vi "Serial-Communication-LabVIEW.vi"() -> ()   [LabVIEW 2016]
uses:
  <vilib>/Instr/_visa.llb/VISA Configure Serial Port (Instr).vi
panel:
  out "O7":bool
  out "O6":bool
  out "O5":bool
  out "O4":bool
  out "O3":bool
  out "O2":bool
  out "O1":bool
  out "O0":bool
  in  "17":bool
  in  "16":bool
  in  "15":bool
  in  "14":bool
  in  "13":bool
  in  "12":bool
  in  "11":bool
  in  "10":bool
  in  "stop":bool
  in  "milliseconds to wait":u32
  in  "VISA resource name":refnum<visa-resource-name>
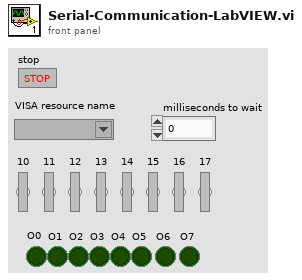
[diagram p1: front panel]
types:
  T1 = cluster{"10":bool, "11":bool, "12":bool, "13":bool, "14":bool, "15":bool, "16":bool, "17":bool}
  T2 = cluster{"Boolean array[0]":bool, "Boolean array[1]":bool, "Boolean array[2]":bool, "Boolean array[3]":bool, "Boolean array[4]":bool, "Boolean array[5]":bool, "Boolean array[6]":bool, "Boolean array[7]":bool, "Boolean array[8]":bool}
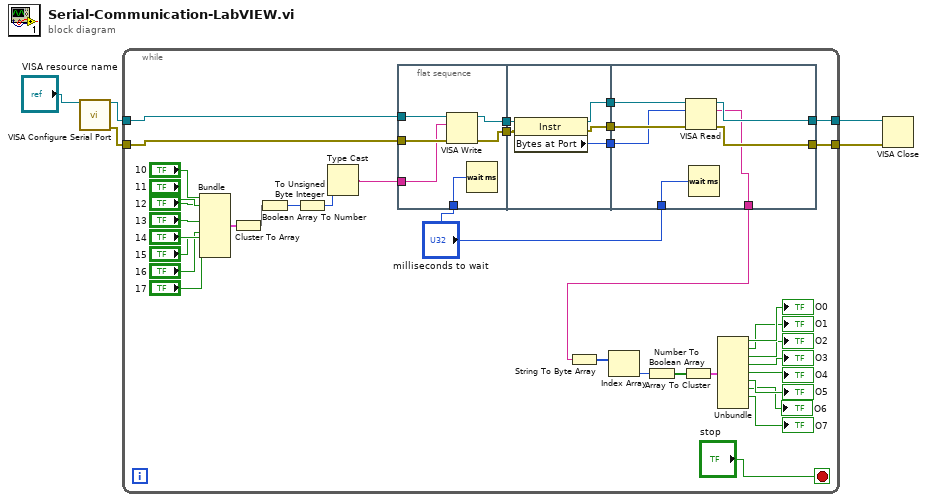
[diagram p0: block diagram]
diagram:
  n1 = call-poly "VISA Configure Serial Port"("VISA resource name"="VISA resource name") -> ("VISA resource name out"=w4:refnum<visa-resource-name>, "error out"=w3:errorcluster)  [unwired: 13 in]
  n2 = while {
    tunnel: w3 -> [w36]
    tunnel: [w34] -> w1
    tunnel: w4 -> [w37]
    tunnel: [w35] -> w2
    stop <- "stop" stop-if-true
    n3 = Bundle("10"="10", "11"="11", "12"="12", "13"="13", "14"="14", "15"="15", "16"="16", "17"="17") -> (w25:T1)  [unwired: 1 in]
    n4 = Cluster To Array(cluster=w25) -> (array=w24:bool[])
    n5 = Boolean Array To Number(Boolean array=w24) -> (number=w23:u32)
    n6 = To Unsigned Byte Integer(number=w23) -> (unsigned 8bit integer=w22:u8)
    n7 = Type Cast(x=w22) -> (*(type *) &x=w21:string)  [unwired: 1 in]
    n8 = flat-sequence {
      tunnel: [w48] -> w42
      tunnel: [w47] -> w41
      tunnel: w37 -> [w46]
      tunnel: w36 -> [w45]
      tunnel: "milliseconds to wait" -> [w44]
      tunnel: w21 -> [w43]
      tunnel: w42 -> [w53]
      tunnel: w41 -> [w52]
      tunnel: [w51] -> w40
      tunnel: [w50] -> w39
      tunnel: [w49] -> w38
      tunnel: w40 -> [w60]
      tunnel: w39 -> [w59]
      tunnel: [w58] -> w35
      tunnel: [w57] -> w34
      tunnel: "milliseconds to wait" -> [w56]
      tunnel: w38 -> [w55]
      tunnel: [w54] -> w20
      frame #0 {
        n9 = VISA Write(VISA resource name=w46, write buffer=w43, error in (no error)=w45) -> (VISA resource name out=w48:refnum<visa-resource-name>, error out=w47:errorcluster)  [unwired: 1 out]
        n10 = Wait (ms)(milliseconds to wait=w44) -> ()  [unwired: 1 out]
      }
      frame #1 {
        n11 = property class="Instr"(reference=w53, error in=w52) -> (reference out=w51:refnum<visa-resource-name>, error out=w50:errorcluster, "Bytes at Port"=w49:u32)
      }
      frame #2 {
        n12 = VISA Read(VISA resource name=w60, byte count=w55, error in (no error)=w59) -> (VISA resource name out=w58:refnum<visa-resource-name>, read buffer=w54:string, error out=w57:errorcluster)  [unwired: 1 out]
        n13 = Wait (ms)(milliseconds to wait=w56) -> ()  [unwired: 1 out]
      }
    }
    n14 = String To Byte Array(string=w20) -> (unsigned byte array=w19:u8[])
    n15 = Index Array(array=w19) -> (element=w18:u8)  [unwired: 1 in]
    n16 = Number To Boolean Array(number=w18) -> (Boolean array=w17:bool[])
    n17 = Array To Cluster(array=w17) -> (cluster=w16:T2)
    n18 = Unbundle(w16) -> ("Boolean array[0]"=→"O0":bool, "Boolean array[1]"=→"O1":bool, "Boolean array[2]"=→"O2":bool, "Boolean array[3]"=→"O3":bool, "Boolean array[4]"=→"O4":bool, "Boolean array[5]"=→"O5":bool, "Boolean array[6]"=→"O6":bool, "Boolean array[7]"=→"O7":bool)  [unwired: 1 out]
  }
  n19 = VISA Close(VISA resource name=w2, error in (no error)=w1) -> ()  [unwired: 1 out]
